vi "API Example - Add1.vi"(10 "input2":dbl=4.0, 11 "input1":dbl=3.0) -> (3 "sum":dbl)   [LabVIEW 2017]
panel:
  out "difference":dbl
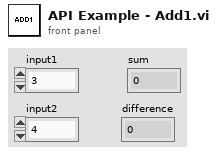
[diagram p1: front panel]
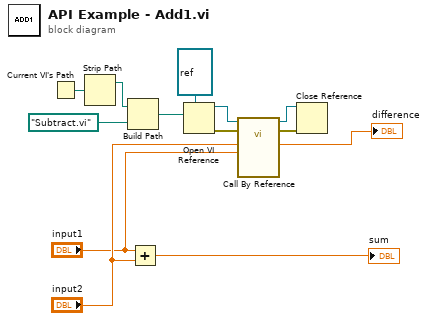
[diagram p0: block diagram]
diagram:
  n1 = Current VI's Path() -> (path=w8:path)
  n2 = Strip Path(path=w8) -> (stripped path=w7:path)  [unwired: 1 out]
  n3 = Build Path(base path=w7, name or relative path=path "Subtract.vi") -> (appended path=w5:path)
  n4 = Add(x="input1", y="input2") -> (x+y=→"sum":dbl)
  n5 = Open VI Reference(type specifier VI Refnum (for type only)=refnum<vi> refnum, vi path=w5) -> (vi reference=w13:refnum<vi>, error out=w12:errorcluster)  [unwired: 1 in, 3 out]
  n6 = call-by-ref "?"(reference=w13, error in=w12, "input2"="input1", "input1"="input2") -> (reference out=w10:refnum<vi>, error out=w11:errorcluster, "output"=→"difference":dbl)  [unwired: 9 in]
  n7 = Close Reference(reference=w10, error in (no error)=w11) -> ()  [unwired: 1 out]
